vi "SBML Information.vi"(0 "Read SBML File":string="<?xml version='1.0' encoding='UTF-8' standalone='no'?>\n<sbml xmlns=\"http://www.sbml.org/sbml/level3/version1/core\" level=\"3\" version=\"1\">\n  <model name=\"Created by iBioSim flatten routine\" volumeUnits=\"litre\" id=\"or\" substanceUnits=\"mole\" metaid=\"iBioSim47\">\n    <listOfUnitDefinitions>\n      <unitDefinition id=\"u_1_second_n1\">\n        <listOfUnits>\n          <unit scale=\"0\" kind=\"second\" multiplier=\"1\" exponent=\"-1\"/>\n        </listOfUnits>\n      </unitDefinition>\n      <unitDefinition id=\"u_1_mole_n1\">\n        <listOfUnits>\n          <unit scale=\"0\" kind=\"mole\" multiplier=\"1\" exponent=\"-1\"/>\n        </listOfUnits>\n      </unitDefinition>\n    </listOfUnitDefinitions>\n    <listOfCompartments>\n      <compartment constant=\"true\" id=\"Cell\" size=\"1\" spatialDimensions=\"3\"/>\n    </listOfCompartments>\n    <listOfSpecies>\n      <species boundaryCondition=\"false\" constant=\"false\" metaid=\"iBioSim31\" hasOnlySubstanceUnits=\"true\" initialAmount=\"0\" compartment=\"Cell\" id=\"CI\"/>\n      <species boundaryCondition=\"false\" constant=\"false\" metaid=\"iBioSim32\" hasOnlySubstanceUnits=\"true\" initialAmount=\"0\" compartment=\"Cell\" id=\"GFP\"/>\n      <species boundaryCondition=\"true\" constant=\"false\" metaid=\"iBioSim33\" hasOnlySubstanceUnits=\"true\" initialAmount=\"0\" compartment=\"Cell\" id=\"LacI\"/>\n      <species boundaryCondition=\"true\" constant=\"false\" metaid=\"iBioSim34\" hasOnlySubstanceUnits=\"true\" initialAmount=\"0\" compartment=\"Cell\" id=\"TetR\"/>\n      <species boundaryCondition=\"false\" constant=\"false\" metaid=\"iBioSim35\" hasOnlySubstanceUnits=\"true\" initialAmount=\"0\" compartment=\"Cell\" id=\"Cro\"/>\n      <species boundaryCondition=\"false\" constant=\"false\" metaid=\"iBioSim36\" hasOnlySubstanceUnits=\"true\" initialAmount=\"2\" sboTerm=\"SBO:0000590\" compartment=\"Cell\" id=\"Promoter_CI\"/>\n      <species boundaryCondition=\"false\" constant=\"false\" metaid=\"iBioSim37\" hasOnlySubstanceUnits=\"true\" initialAmount=\"2\" sboTerm=\"SBO:0000590\" compartment=\"Cell\" id=\"Promoter_Cro\"/>\n      <species boundaryCondition=\"false\" constant=\"false\" metaid=\"iBioSim38\" hasOnlySubstanceUnits=\"true\" initialAmount=\"2\" sboTerm=\"SBO:0000590\" compartment=\"Cell\" id=\"P1\"/>\n      <species boundaryCondition=\"false\" constant=\"false\" metaid=\"iBioSim39\" hasOnlySubstanceUnits=\"true\" initialAmount=\"2\" sboTerm=\"SBO:0000590\" compartment=\"Cell\" id=\"P2\"/>\n    </listOfSpecies>\n    <listOfParameters>\n      <parameter name=\"Reverse RNAP binding rate\" constant=\"true\" id=\"ko_r\" metaid=\"iBioSim2\" value=\"1\"/>\n      <parameter name=\"Initial RNAP count\" constant=\"true\" id=\"nr\" metaid=\"iBioSim7\" value=\"30\"/>\n      <parameter name=\"Stoichiometry of production\" constant=\"true\" id=\"np\" metaid=\"iBioSim8\" value=\"10\"/>\n      <parameter name=\"Reverse repression binding rate\" constant=\"true\" id=\"kr_r\" metaid=\"iBioSim9\" value=\"1\"/>\n      <parameter name=\"Forward activation binding rate\" constant=\"true\" id=\"ka_f\" metaid=\"iBioSim10\" value=\"0.0033\"/>\n      <parameter name=\"Extracellular diffusion rate\" constant=\"true\" id=\"kecdiff\" metaid=\"iBioSim11\" value=\"1\"/>\n      <parameter name=\"Open complex production rate\" constant=\"true\" id=\"ko\" metaid=\"iBioSim12\" value=\"0.05\"/>\n      <parameter name=\"Forward membrane diffusion rate\" constant=\"true\" id=\"kmdiff_f\" metaid=\"iBioSim13\" value=\"1\"/>\n      <parameter name=\"Extracellular degradation rate\" constant=\"true\" id=\"kecd\" metaid=\"iBioSim14\" value=\"0.005\"/>\n      <parameter name=\"Reverse complex formation rate\" constant=\"true\" id=\"kc_r\" metaid=\"iBioSim15\" value=\"1\"/>\n      <parameter name=\"Forward repression binding rate\" constant=\"true\" id=\"kr_f\" metaid=\"iBioSim16\" value=\"0.5\"/>\n      <parameter name=\"Reverse activation binding rate\" constant=\"true\" id=\"ka_r\" metaid=\"iBioSim17\" value=\"1\"/>\n      <parameter name=\"Stoichiometry of binding\" constant=\"true\" id=\"nc\" metaid=\"iBioSim18\" value=\"2\"/>\n      <parameter name=\"Reverse activated RNAP binding rate\" constant=\"true\" id=\"kao_r\" metaid=\"iBioSim19\" value=\"1\"/>\n      <parameter name=\"Degradation rate\" constant=\"true\" id=\"kd\" metaid=\"iBioSim20\" value=\"0.0075\"/>\n      <parameter name=\"Basal production rate\" constant=\"true\" id=\"kb\" metaid=\"iBioSim21\" value=\"0.0001\"/>\n      <parameter name=\"Initial promoter count\" constant=\"true\" id=\"ng\" metaid=\"iBioSim22\" value=\"2\"/>\n      <parameter name=\"Activated production rate\" constant=\"true\" id=\"ka\" metaid=\"iBioSim23\" value=\"0.25\"/>\n      <parameter name=\"Forward activated RNAP binding rate\" constant=\"true\" id=\"kao_f\" metaid=\"iBioSim24\" value=\"1\"/>\n      <parameter name=\"Reverse membrane diffusion rate\" constant=\"true\" id=\"kmdiff_r\" metaid=\"iBioSim25\" value=\"0.01\"/>\n      <parameter name=\"Forward RNAP binding rate\" constant=\"true\" id=\"ko_f\" metaid=\"iBioSim26\" value=\"0.033\"/>\n      <parameter name=\"Forward complex formation rate\" constant=\"true\" id=\"kc_f\" metaid=\"iBioSim27\" value=\"0.05\"/>\n      <parameter constant=\"true\" id=\"High\" metaid=\"iBioSim28\" value=\"120\"/>\n      <parameter constant=\"true\" id=\"HighTime\" metaid=\"iBioSim29\" value=\"2000\"/>\n      <parameter constant=\"true\" id=\"HighTime2\" metaid=\"iBioSim30\" value=\"4000\"/>\n    </listOfParameters>\n    <listOfReactions>\n      <reaction compartment=\"Cell\" fast=\"false\" id=\"Degradation_GFP\" reversible=\"false\">\n        <listOfReactants>\n          <speciesReference stoichiometry=\"1\" constant=\"true\" species=\"GFP\"/>\n        </listOfReactants>\n        <kineticLaw>\n          <math xmlns=\"http://www.w3.org/1998/Math/MathML\">          \n            <apply>\n              <times/>\n              <ci> kd </ci>\n              <ci> GFP </ci>\n            </apply>\n          </math>\n                  <listOfLocalParameters>\n            <localParameter id=\"kd\" units=\"u_1_second_n1\" value=\"0.0075\"/>\n          </listOfLocalParameters>\n        </kineticLaw>\n      </reaction>\n      <reaction compartment=\"Cell\" fast=\"false\" id=\"Degradation_Cro\" reversible=\"false\">\n        <listOfReactants>\n          <speciesReference stoichiometry=\"1\" constant=\"true\" species=\"Cro\"/>\n        </listOfReactants>\n        <kineticLaw>\n          <math xmlns=\"http://www.w3.org/1998/Math/MathML\">          \n            <apply>\n              <times/>\n              <ci> kd </ci>\n              <ci> Cro </ci>\n            </apply>\n          </math>\n                  <listOfLocalParameters>\n            <localParameter id=\"kd\" units=\"u_1_second_n1\" value=\"0.0075\"/>\n          </listOfLocalParameters>\n        </kineticLaw>\n      </reaction>\n      <reaction compartment=\"Cell\" fast=\"false\" id=\"Degradation_CI\" reversible=\"false\">\n        <listOfReactants>\n          <speciesReference stoichiometry=\"1\" constant=\"true\" species=\"CI\"/>\n        </listOfReactants>\n        <kineticLaw>\n          <math xmlns=\"http://www.w3.org/1998/Math/MathML\">          \n            <apply>\n              <times/>\n              <ci> kd </ci>\n              <ci> CI </ci>\n            </apply>\n          </math>\n                  <listOfLocalParameters>\n            <localParameter id=\"kd\" units=\"u_1_second_n1\" value=\"0.0075\"/>\n          </listOfLocalParameters>\n        </kineticLaw>\n      </reaction>\n      <reaction compartment=\"Cell\" fast=\"false\" id=\"Degradation_TetR\" reversible=\"false\">\n        <listOfReactants>\n          <speciesReference stoichiometry=\"1\" constant=\"true\" species=\"TetR\"/>\n        </listOfReactants>\n        <kineticLaw>\n          <math xmlns=\"http://www.w3.org/1998/Math/MathML\">          \n            <apply>\n              <times/>\n              <ci> kd </ci>\n              <ci> TetR </ci>\n            </apply>\n          </math>\n                  <listOfLocalParameters>\n            <localParameter id=\"kd\" units=\"u_1_second_n1\" value=\"0.0075\"/>\n          </listOfLocalParameters>\n        </kineticLaw>\n      </reaction>\n      <reaction compartment=\"Cell\" fast=\"false\" id=\"Degradation_LacI\" reversible=\"false\">\n        <listOfReactants>\n          <speciesReference stoichiometry=\"1\" constant=\"true\" species=\"LacI\"/>\n        </listOfReactants>\n        <kineticLaw>\n          <math xmlns=\"http://www.w3.org/1998/Math/MathML\">          \n            <apply>\n              <times/>\n              <ci> kd </ci>\n              <ci> LacI </ci>\n            </apply>\n          </math>\n                  <listOfLocalParameters>\n            <localParameter id=\"kd\" units=\"u_1_second_n1\" value=\"0.0075\"/>\n          </listOfLocalParameters>\n        </kineticLaw>\n      </reaction>\n      <reaction compartment=\"Cell\" fast=\"false\" id=\"R_abstracted_production_Promoter_CI\" reversible=\"false\">\n        <listOfProducts>\n          <speciesReference stoichiometry=\"10\" constant=\"true\" species=\"CI\"/>\n        </listOfProducts>\n        <listOfModifiers>\n          <modifierSpeciesReference species=\"LacI\"/>\n        </listOfModifiers>\n        <kineticLaw>\n          <math xmlns=\"http://www.w3.org/1998/Math/MathML\">          \n            <apply>\n              <divide/>\n              <apply>\n                <times/>\n                <apply>\n                  <times/>\n                  <ci> ko__Promoter_CI </ci>\n                  <ci> ng__Promoter_CI </ci>\n                </apply>\n                <apply>\n                  <times/>\n                  <ci> Ko__Promoter_CI </ci>\n                  <ci> RNAP </ci>\n                </apply>\n              </apply>\n              <apply>\n                <plus/>\n                <apply>\n                  <plus/>\n                  <cn type=\"integer\"> 1 </cn>\n                  <apply>\n                    <times/>\n                    <ci> Ko__Promoter_CI </ci>\n                    <ci> RNAP </ci>\n                  </apply>\n                </apply>\n                <apply>\n                  <power/>\n                  <apply>\n                    <times/>\n                    <ci> Kr__LacI_Promoter_CI </ci>\n                    <ci> LacI </ci>\n                  </apply>\n                  <ci> nc__LacI_Promoter_CI </ci>\n                </apply>\n              </apply>\n            </apply>\n          </math>\n                  <listOfLocalParameters>\n            <localParameter id=\"RNAP\" units=\"u_1_mole_n1\" value=\"30\"/>\n            <localParameter id=\"ng__Promoter_CI\" units=\"u_1_mole_n1\" value=\"2\"/>\n            <localParameter id=\"Ko__Promoter_CI\" units=\"u_1_mole_n1\" value=\"0.033\"/>\n            <localParameter id=\"ko__Promoter_CI\" units=\"u_1_second_n1\" value=\"0.05\"/>\n            <localParameter id=\"nc__LacI_Promoter_CI\" units=\"dimensionless\" value=\"2\"/>\n            <localParameter id=\"Kr__LacI_Promoter_CI\" units=\"u_1_mole_n1\" value=\"0.5\"/>\n          </listOfLocalParameters>\n        </kineticLaw>\n      </reaction>\n      <reaction compartment=\"Cell\" fast=\"false\" id=\"R_abstracted_production_P1\" reversible=\"false\">\n        <listOfProducts>\n          <speciesReference stoichiometry=\"10\" constant=\"true\" species=\"GFP\"/>\n        </listOfProducts>\n        <listOfModifiers>\n          <modifierSpeciesReference species=\"CI\"/>\n        </listOfModifiers>\n        <kineticLaw>\n          <math xmlns=\"http://www.w3.org/1998/Math/MathML\">          \n            <apply>\n              <divide/>\n              <apply>\n                <times/>\n                <apply>\n                  <times/>\n                  <ci> ko__P1 </ci>\n                  <ci> ng__P1 </ci>\n                </apply>\n                <apply>\n                  <times/>\n                  <ci> Ko__P1 </ci>\n                  <ci> RNAP </ci>\n                </apply>\n              </apply>\n              <apply>\n                <plus/>\n                <apply>\n                  <plus/>\n                  <cn type=\"integer\"> 1 </cn>\n                  <apply>\n                    <times/>\n                    <ci> Ko__P1 </ci>\n                    <ci> RNAP </ci>\n                  </apply>\n                </apply>\n                <apply>\n                  <power/>\n                  <apply>\n                    <times/>\n                    <ci> Kr__CI_P1 </ci>\n                    <ci> CI </ci>\n                  </apply>\n                  <ci> nc__CI_P1 </ci>\n                </apply>\n              </apply>\n            </apply>\n          </math>\n                  <listOfLocalParameters>\n            <localParameter id=\"RNAP\" units=\"u_1_mole_n1\" value=\"30\"/>\n            <localParameter id=\"ng__P1\" units=\"u_1_mole_n1\" value=\"2\"/>\n            <localParameter id=\"Ko__P1\" units=\"u_1_mole_n1\" value=\"0.033\"/>\n            <localParameter id=\"ko__P1\" units=\"u_1_second_n1\" value=\"0.05\"/>\n            <localParameter id=\"nc__CI_P1\" units=\"dimensionless\" value=\"2\"/>\n            <localParameter id=\"Kr__CI_P1\" units=\"u_1_mole_n1\" value=\"0.5\"/>\n          </listOfLocalParameters>\n        </kineticLaw>\n      </reaction>\n      <reaction compartment=\"Cell\" fast=\"false\" id=\"R_abstracted_production_P2\" reversible=\"false\">\n        <listOfProducts>\n          <speciesReference stoichiometry=\"10\" constant=\"true\" species=\"GFP\"/>\n        </listOfProducts>\n        <listOfModifiers>\n          <modifierSpeciesReference species=\"Cro\"/>\n        </listOfModifiers>\n        <kineticLaw>\n          <math xmlns=\"http://www.w3.org/1998/Math/MathML\">          \n            <apply>\n              <divide/>\n              <apply>\n                <times/>\n                <apply>\n                  <times/>\n                  <ci> ko__P2 </ci>\n                  <ci> ng__P2 </ci>\n                </apply>\n                <apply>\n                  <times/>\n                  <ci> Ko__P2 </ci>\n                  <ci> RNAP </ci>\n                </apply>\n              </apply>\n              <apply>\n                <plus/>\n                <apply>\n                  <plus/>\n                  <cn type=\"integer\"> 1 </cn>\n                  <apply>\n                    <times/>\n                    <ci> Ko__P2 </ci>\n                    <ci> RNAP </ci>\n                  </apply>\n                </apply>\n                <apply>\n                  <power/>\n                  <apply>\n                    <times/>\n                    <ci> Kr__Cro_P2 </ci>\n                    <ci> Cro </ci>\n                  </apply>\n                  <ci> nc__Cro_P2 </ci>\n                </apply>\n              </apply>\n            </apply>\n          </math>\n                  <listOfLocalParameters>\n            <localParameter id=\"RNAP\" units=\"u_1_mole_n1\" value=\"30\"/>\n            <localParameter id=\"ng__P2\" units=\"u_1_mole_n1\" value=\"2\"/>\n            <localParameter id=\"Ko__P2\" units=\"u_1_mole_n1\" value=\"0.033\"/>\n            <localParameter id=\"ko__P2\" units=\"u_1_second_n1\" value=\"0.05\"/>\n            <localParameter id=\"nc__Cro_P2\" units=\"dimensionless\" value=\"2\"/>\n            <localParameter id=\"Kr__Cro_P2\" units=\"u_1_mole_n1\" value=\"0.5\"/>\n          </listOfLocalParameters>\n        </kineticLaw>\n      </reaction>\n      <reaction compartment=\"Cell\" fast=\"false\" id=\"R_abstracted_production_Promoter_Cro\" reversible=\"false\">\n        <listOfProducts>\n          <speciesReference stoichiometry=\"10\" constant=\"true\" species=\"Cro\"/>\n        </listOfProducts>\n        <listOfModifiers>\n          <modifierSpeciesReference species=\"TetR\"/>\n        </listOfModifiers>\n        <kineticLaw>\n          <math xmlns=\"http://www.w3.org/1998/Math/MathML\">          \n            <apply>\n              <divide/>\n              <apply>\n                <times/>\n                <apply>\n                  <times/>\n                  <ci> ko__Promoter_Cro </ci>\n                  <ci> ng__Promoter_Cro </ci>\n                </apply>\n                <apply>\n                  <times/>\n                  <ci> Ko__Promoter_Cro </ci>\n                  <ci> RNAP </ci>\n                </apply>\n              </apply>\n              <apply>\n                <plus/>\n                <apply>\n                  <plus/>\n                  <cn type=\"integer\"> 1 </cn>\n                  <apply>\n                    <times/>\n                    <ci> Ko__Promoter_Cro </ci>\n                    <ci> RNAP </ci>\n                  </apply>\n                </apply>\n                <apply>\n                  <power/>\n                  <apply>\n                    <times/>\n                    <ci> Kr__TetR_Promoter_Cro </ci>\n                    <ci> TetR </ci>\n                  </apply>\n                  <ci> nc__TetR_Promoter_Cro </ci>\n                </apply>\n              </apply>\n            </apply>\n          </math>\n                  <listOfLocalParameters>\n            <localParameter id=\"RNAP\" units=\"u_1_mole_n1\" value=\"30\"/>\n            <localParameter id=\"ng__Promoter_Cro\" units=\"u_1_mole_n1\" value=\"2\"/>\n            <localParameter id=\"Ko__Promoter_Cro\" units=\"u_1_mole_n1\" value=\"0.033\"/>\n            <localParameter id=\"ko__Promoter_Cro\" units=\"u_1_second_n1\" value=\"0.05\"/>\n            <localParameter id=\"nc__TetR_Promoter_Cro\" units=\"dimensionless\" value=\"2\"/>\n            <localParameter id=\"Kr__TetR_Promoter_Cro\" units=\"u_1_mole_n1\" value=\"0.5\"/>\n          </listOfLocalParameters>\n        </kineticLaw>\n      </reaction>\n    </listOfReactions>\n    <listOfEvents>\n      <event id=\"event0\" metaid=\"iBioSim45\" useValuesFromTriggerTime=\"true\">\n        <trigger persistent=\"true\" initialValue=\"true\">\n          <math xmlns=\"http://www.w3.org/1998/Math/MathML\">          \n            <apply>\n              <geq/>\n              <csymbol encoding=\"text\" definitionURL=\"http://www.sbml.org/sbml/symbols/time\"> t </csymbol>\n              <ci> HighTime </ci>\n            </apply>\n          </math>\n                </trigger>\n        <listOfEventAssignments>\n          <eventAssignment variable=\"TetR\">\n            <math xmlns=\"http://www.w3.org/1998/Math/MathML\">            \n              <ci> High </ci>\n            </math>\n                    </eventAssignment>\n        </listOfEventAssignments>\n      </event>\n      <event id=\"event1\" metaid=\"iBioSim46\" useValuesFromTriggerTime=\"true\">\n        <trigger persistent=\"true\" initialValue=\"true\">\n          <math xmlns=\"http://www.w3.org/1998/Math/MathML\">          \n            <apply>\n              <geq/>\n              <csymbol encoding=\"text\" definitionURL=\"http://www.sbml.org/sbml/symbols/time\"> t </csymbol>\n              <ci> HighTime2 </ci>\n            </apply>\n          </math>\n                </trigger>\n        <listOfEventAssignments>\n          <eventAssignment variable=\"LacI\">\n            <math xmlns=\"http://www.w3.org/1998/Math/MathML\">            \n              <ci> High </ci>\n            </math>\n                    </eventAssignment>\n        </listOfEventAssignments>\n      </event>\n    </listOfEvents>\n  </model>\n</sbml>", 11 "error in (no error)":errorcluster) -> (4 "Level":string, 6 "Version":string, 8 "Model Name":string, 10 "ID":string, 15 "error out":errorcluster)   [LabVIEW 2014]
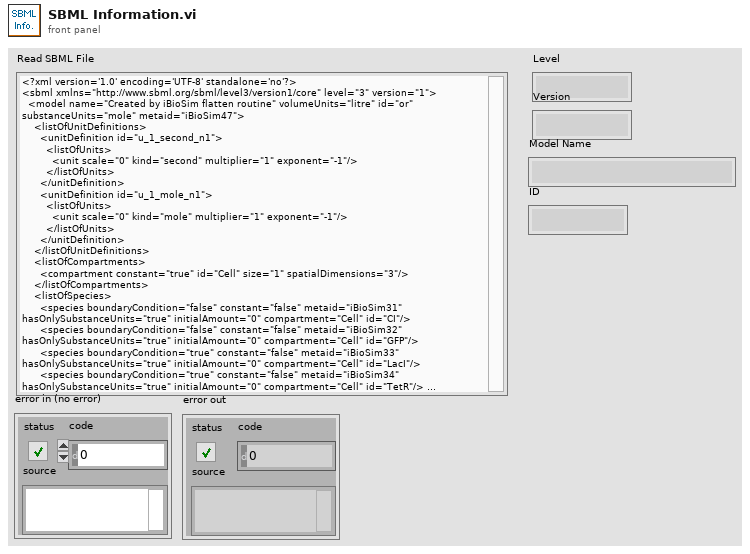
[diagram p1: front panel]
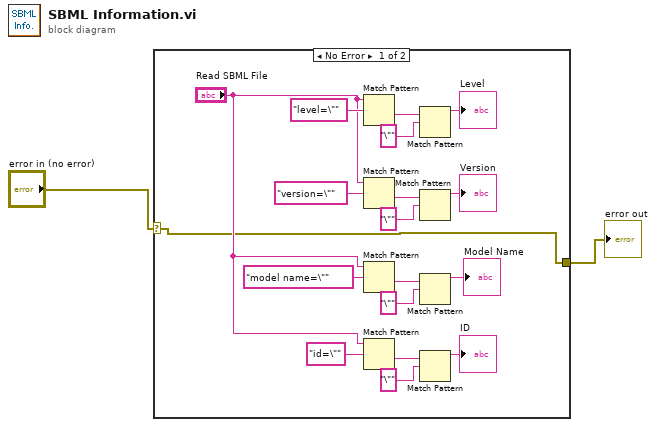
[diagram p0: block diagram]
diagram:
  n1 = case shown="No Error" "error in (no error)" {
    selector: "error in (no error)" -> [w3 w21]
    tunnel: [w3 w21] -> w1
    frame No Error {
      n2 = Match Pattern(string="Read SBML File", regular expression="level=\"") -> (after substring=w19:string)  [unwired: 1 in, 3 out]
      n3 = Match Pattern(string="Read SBML File", regular expression="version=\"") -> (after substring=w15:string)  [unwired: 1 in, 3 out]
      n4 = Match Pattern(string="Read SBML File", regular expression="model name=\"") -> (after substring=w11:string)  [unwired: 1 in, 3 out]
      n5 = Match Pattern(string="Read SBML File", regular expression="id=\"") -> (after substring=w7:string)  [unwired: 1 in, 3 out]
      n6 = Match Pattern(string=w19, regular expression="\"") -> (before substring=→"Level":string)  [unwired: 1 in, 3 out]
      n7 = Match Pattern(string=w15, regular expression="\"") -> (before substring=→"Version":string)  [unwired: 1 in, 3 out]
      n8 = Match Pattern(string=w11, regular expression="\"") -> (before substring=→"Model Name":string)  [unwired: 1 in, 3 out]
      n9 = Match Pattern(string=w7, regular expression="\"") -> (before substring=→"ID":string)  [unwired: 1 in, 3 out]
    }
    frame Error {
    }
  }
  "error out" <- w1
